vi "Add Data Replay RTM Dependency.vi"(8 "error in (no error)":errorcluster, 9 "Menu hierarchy in":string[](array[string]), 11 "Node Ptr":u64 format="%.0x") -> (0 "error out":errorcluster, 1 "Menu hierarchy out":string[](array[string]), 3 "Action":T1)   [LabVIEW 2011, in "Engine Sim System Explorer.lvlib"]
uses:
  Engine Sim System Explorer.lvlib
  <vilib>/NI Veristand/Custom Device API/Custom Device RTM Dependency.ctl
  <vilib>/NI Veristand/Custom Device API/Custom Device API.lvlib
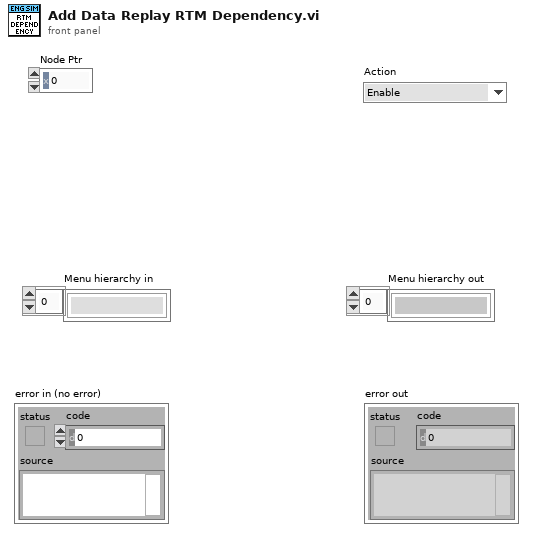
[diagram p1: front panel]
types:
  T1 = typedef "Custom Device API.lvlib/Custom Device RTM Dependency.ctl" = enum16{"Enable", "Disable", "Hide"}
  T2 = typedef "Custom Device API.lvlib/Custom Device Item Ref.ctl" = u64
  T3 = typedef "Engine Sim System Explorer.lvlib/DataReplayComp.ctl" = cluster{"Name":string, "Number":i32, "Optionals":bool[]}
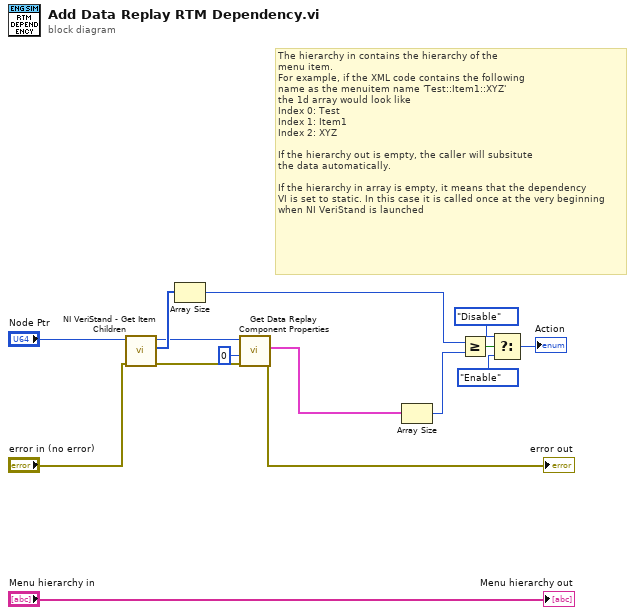
[diagram p0: block diagram]
diagram:
  # "The hierarchy in contains the hierarchy of the\nmenu item.\nFor example, if the XML code contains the following\nname as the menuitem name 'Test::Item1::XYZ'\nthe 1d array would look like\nIndex 0: Test\nIndex 1: Item1\nIndex 2: XYZ\n\nIf the hierarchy out is empty, the caller will subsitute\nthe data automatically.\n\nIf the hierarchy in array is empty, it means that the dependency\nVI is set to static. In this case it is called once at the very beginning\nwhen NI VeriStand is launched"
  n1 = call <vilib>:"NI VeriStand - Get Item Children.vi"("error in (no error)"="error in (no error)", "Item Ref in"="Node Ptr") -> ("error out"=w12:errorcluster, "Child Refs"=w14:T2[], "Item Ref out"=w13:T2)  [unwired: 6 in, 1 out]
  n2 = Array Size(array=w14) -> (size(s)=w11:i32)
  n3 = call "Get Data Replay Component Properties.vi"("error in (no error)"=w12, "Prefix #"=0, "Item Ref in"=w13) -> ("error out"=→"error out":errorcluster, "DataReplays"=w2:T3[])  [unwired: 6 in, 1 out]
  n4 = Array Size(array=w2) -> (size(s)=w7:i32)
  n5 = Greater Or Equal?(x=w11, y=w7) -> (x >= y?=w10:bool)
  n6 = Select(t=Custom_Device_RTM_Dependency."Disable" ("Action"), s=w10, f=Custom_Device_RTM_Dependency."Enable" ("Action")) -> (s? t:f=→"Action":T1)
  "Menu hierarchy out" <- "Menu hierarchy in"
